vi "Controller Generate Filter Coefficients From Transfer Function.vi"(4 "Destination Folder":path, 5 "iwl coeff b":i16=2, 6 "Filter Name":string, 7 "iwl coeff a":i16=2, 8 "Generate FPGA Code?":bool, 9 "wl":i16=20, 10 "denominator":dbl[](array[numeric]), 11 "numerator":dbl[](array[numeric])) -> (1 "gain":dbl, 2 "coeff a":dbl[](array[numeric]), 3 "coeff b":dbl[](array[numeric]))   [LabVIEW 2011, in "Controller VIs.lvlib"]
uses:
  Controller VIs.lvlib
  <vilib>/addons/Digital Filter Design/_Objects.llb/DFD Output Iwl Obj.ctl
  <vilib>/addons/Digital Filter Design/_Objects.llb/DFD Quantization Settings.ctl
  <vilib>/addons/Digital Filter Design/_Objects.llb/DFD Quantization Sources.ctl
  <vilib>/addons/Digital Filter Design/_Objects.llb/DFD Phase Setting.ctl
  <vilib>/addons/Digital Filter Design/_Objects.llb/DFD Coef Norm Type.ctl
  <vilib>/addons/Digital Filter Design/FXPModel.llb/DFD FXP Quantize Coef (Advanced).vi
  <vilib>/addons/Digital Filter Design/NI_DigFilterLicensed.lvlib
  <vilib>/addons/Digital Filter Design/CodeGen.llb/DFD FXP LabVIEW FPGA Code Generator.vi
panel:
  out "max gain error (dB)":dbl
  out "max phase error (deg)":dbl
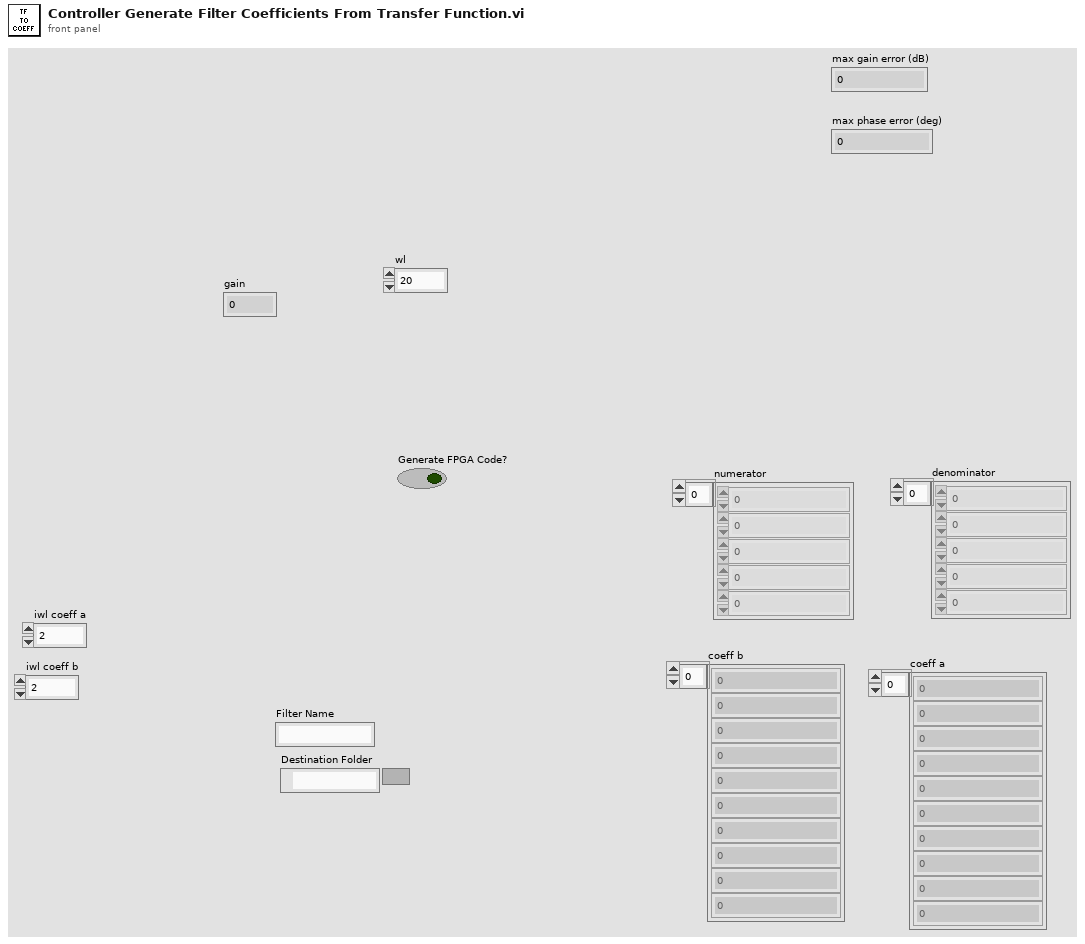
[diagram p1: front panel]
types:
  T1 = typedef "NI_DigFilterLicensed.lvlib/DFD Coef Norm Type.ctl" = enum16{"No Norm", "Time Domain 1-Norm", "Time Domain 2-Norm", "Time Domain Inf-Norm"}
  T2 = typedef "NI_DigFilterLicensed.lvlib/DFD Phase Setting.ctl" = cluster{"unwrap? (F)":bool, "degree? (F)":bool}
  T3 = typedef "NI_DigFilterLicensed.lvlib/DFD Quantization Settings.ctl" = cluster{"source":T4, "wl":i16, "iwl":i16, "overflow mode":enum16{"Saturation", "Wrap"}, "rounding mode":enum16{"Nearest", "Truncation"}, "signed?":bool}
  T4 = typedef "NI_DigFilterLicensed.lvlib/DFD Quantization Sources.ctl" = u16
  T5 = typedef "NI_DigFilterLicensed.lvlib/DFD Output Iwl Obj.ctl" = cluster{"output option":enum16{"Auto", "Same As Input", "User Defined"}, "integer word length":i16}
  T6 = typedef "NI_DigFilterLicensed.lvlib/DFD Filter Obj.ctl" = cluster{"mSRate_Fs":dbl, "mSRate_Version":string, "mSRate_Comments":string, "mSRate_OrgCoef":T7, "mSRate_CurCoef":T7, "mSRate_Quantized?":bool, "mSRate_QCoef":T7, "mSRate_QSettings":T9[], "mSRate_Order":i32, "mSRate_Scaling":cluster{"mSRate_ScaleByPowerOf2?":bool, "mSRate_ScaleType":T1}}
  T7 = typedef "NI_DigFilterLicensed.lvlib/DFD Filter Coef.ctl" = cluster{"type":T8, "gain":dbl, "coef a (k)":dbl[], "coef b (v)":dbl[]}
  T8 = typedef "NI_DigFilterLicensed.lvlib/DFD Filter Structure Type Selector.ctl" = enum16{"Undefined", "FIR Direct Form", "FIR Direct Form Transposed", "FIR Symmetric", "FIR Antisymmetric", "IIR Direct Form I", "IIR Direct Form I Transposed", "IIR Direct Form II", "IIR Direct Form II Transposed", "IIR Cascaded Second Order Sections Form I", "IIR Cascaded Second Order Sections Form I Transposed", "IIR Cascaded Second Order Sections Form II", "IIR Cascaded Second Order Sections Form II Transposed", "Lattice Allpass (basic sections)", "Lattice Allpass (one multiplier sections)", "Lattice Allpass (normalized sections)", "Lattice AR (basic sections)", "Lattice AR (one multiplier sections)", "Lattice AR (normalized sections)", "Lattice MA (minimum phase)", "Lattice MA (maximum phase)", "Lattice ARMA (basic sections)", "Lattice ARMA (one multiplier sections)", "Lattice ARMA (normalized sections)"}
  T9 = typedef "NI_DigFilterLicensed.lvlib/dfd_Internal Quantization Settings.ctl" = cluster{"source":T10, "wl":i16, "iwl":i16, "overflow mode":enum16{"Saturation", "Wrap"}, "rounding mode":enum16{"Nearest", "Truncation"}, "signed?":bool}
  T10 = typedef "NI_DigFilterLicensed.lvlib/dfd_Internal Quantization Srcs.ctl" = u16
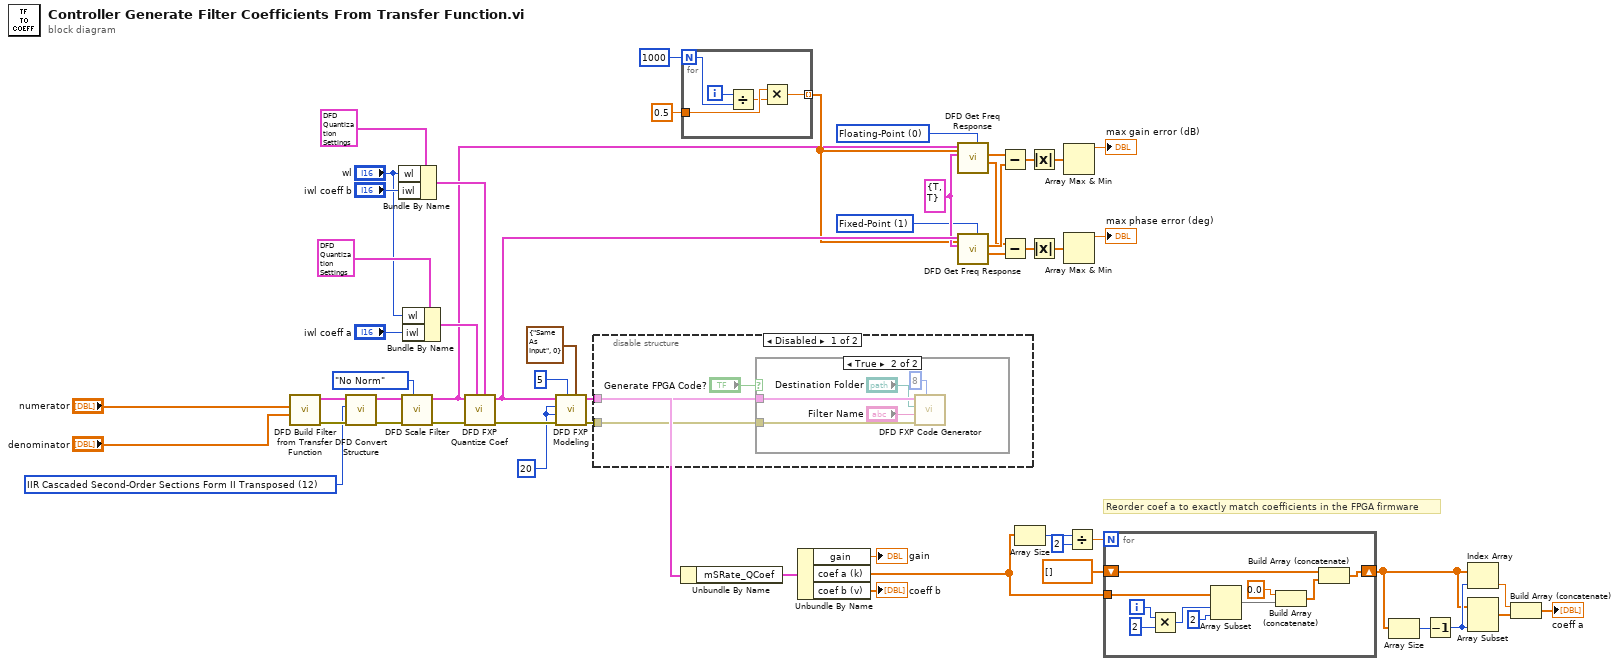
[diagram p0: block diagram]
diagram:
  w32 = u16 0 items=["Floating-Point", "Fixed-Point"] ("output option")
  w40 = u16 1 items=["Floating-Point", "Fixed-Point"] ("output option")
  w41 = T2 {"unwrap? (F)"=TRUE, "degree? (F)"=TRUE} ("phase view")
  w45 = i16 20 ("input word length")
  w52 = u16 12 items=["FIR Direct Form"=1, "FIR Direct Form Transposed"=2, "FIR Symmetric"=3, "FIR Antisymmetric"=4, "IIR Direct Form I"=5, "IIR Direct Form I Transposed"=6, "IIR Direct Form II"=7, "IIR Direct Form II Transposed"=8, "IIR Cascaded Second-Order Sections Form I"=9, "IIR Cascaded Second-Order Sections Form I Transposed"=10, "IIR Cascaded Second-Order Sections Form II"=11, "IIR Cascaded Second-Order Sections Form II Transposed"=12, "Lattice Allpass (basic sections)"=13, "Lattice Allpass (one multiplier sections)"=14, "Lattice Allpass (normalized sections)"=15, "Lattice AR (basic sections)"=16, "Lattice AR (one multiplier sections)"=17, "Lattice AR (normalized sections)"=18, "Lattice MA (minimum phase)"=19, "Lattice MA (maximum phase)"=20, "Lattice ARMA (basic sections)"=21, "Lattice ARMA (one multiplier sections)"=22, "Lattice ARMA (normalized sections)"=23] ("target structure")
  # "Reorder coef a to exactly match coefficients in the FPGA firmware"
  n1 = call <vilib>:"DFD Build Filter from Transfer Function.vi"("denominator"="denominator", "numerator"="numerator") -> ("error out"=w53:errorcluster, "filter out"=w47:T6)  [unwired: 8 in]
  n2 = call <vilib>:"DFD Convert Structure.vi"("error in (no error)"=w53, "target structure"=w52, "filter in"=w47) -> ("error out"=w18:errorcluster, "filter out"=w19:T6)  [unwired: 7 in]
  n3 = Bundle By Name(cluster=T3 {"source"=7, "wl"=20, "iwl"=1, "overflow mode"=enum."Saturation", "rounding mode"=enum."Nearest", "signed?"=TRUE} ("coefficients b/v quantizer"), "wl"="wl", "iwl"="iwl coeff b") -> (w34:T3)
  n4 = call <vilib>:"DFD Scale Filter.vi"("scale type"=DFD_Coef_Norm_Type."No Norm", "error in (no error)"=w18, "filter in"=w19) -> ("error out"=w17:errorcluster, "filter out"=w16:T6)  [unwired: 7 in]
  n5 = Bundle By Name(cluster=T3 {"source"=0, "wl"=20, "iwl"=1, "overflow mode"=enum."Saturation", "rounding mode"=enum."Nearest", "signed?"=TRUE} ("coefficients a/k quantizer"), "wl"="wl", "iwl"="iwl coeff a") -> (w33:T3)
  n6 = call-poly <vilib>:"DFD FXP Quantize Coef.vi"("coefficients b/v quantizer"=w34, "coefficients a/k quantizer"=w33, "error in (no error)"=w17, "filter in"=w16) -> ("error out"=w51:errorcluster, "filter out"=w42:T6)  [unwired: 6 in]
  n7 = call <vilib>:"DFD FXP Modeling.vi"("output integer word length"=T5 {"output option"=enum."Same As Input", "integer word length"=0}, "input integer word length"=i16 5, "error in (no error)"=w51, "output word length"=w45, "input word length"=w45, "filter in"=w42) -> ("error out"=w54:errorcluster, "filter out"=w43:T6)  [unwired: 4 in]
  n8 = disable-structure shown="Disabled" {
    disable-tunnel: w54 -> [w57 _]
    disable-tunnel: w43 -> [w56 _]
    frame Disabled {
      n9 = case shown="True" "Generate FPGA Code?" {
        tunnel: w57 -> [_ w62]
        tunnel: w56 -> [_ w61]
        frame False {
        }
        frame True {
          n10 = call-poly <vilib>:"DFD FXP Code Generator.vi"("# channels"=8, "error in (no error)"=w62, "filter name"="Filter Name", "destination folder"="Destination Folder", "filter in"=w61) -> ()  [unwired: 2 in, 5 out]
        }
      }
    }
    frame Enabled {
    }
  }
  n11 = Unbundle By Name(w43) -> ("mSRate_QCoef"=w50:T7)
  n12 = for {
    N: 1000 -> [w66]
    tunnel: 0.5 -> [w65]
    tunnel: [w63] -> w27 mode=indexing
    i -> [w67]
    n13 = Divide(x=w67, y=w66) -> (x/y=w64:dbl)
    n14 = Multiply(x=w65, y=w64) -> (x*y=w63:dbl)
  }
  n15 = Unbundle By Name(w50) -> ("gain"=→"gain":dbl, "coef a (k)"=w11:dbl[], "coef b (v)"=→"coeff b":dbl[])
  n16 = call <vilib>:"DFD Get Freq Response.vi"("output option"=w32, "freq points [Hz]"=w27, "phase view"=w41, "filter in"=w16) -> ("phase"=w29:dbl[], "magnitude"=w31:dbl[])  [unwired: 4 in, 2 out]
  n17 = call <vilib>:"DFD Get Freq Response.vi"("output option"=w40, "freq points [Hz]"=w27, "phase view"=w41, "filter in"=w42) -> ("phase"=w28:dbl[], "magnitude"=w30:dbl[])  [unwired: 4 in, 2 out]
  n18 = Subtract(x=w31, y=w30) -> (x-y=w25:dbl[])
  n19 = Subtract(x=w29, y=w28) -> (x-y=w22:dbl[])
  n20 = Array Size(array=w11) -> (size(s)=w10:i32)
  n21 = Absolute Value(x=w25) -> (abs(x)=w24:dbl[])
  n22 = Absolute Value(x=w22) -> (abs(x)=w23:dbl[])
  n23 = Array Max & Min(array=w24) -> (max value=→"max gain error (dB)":dbl)  [unwired: 3 out]
  n24 = Array Max & Min(array=w23) -> (max value=→"max phase error (deg)":dbl)  [unwired: 3 out]
  n25 = Divide(x=w10, y=2) -> (x/y=w13:dbl)
  n26 = for {
    N: w13 -> [_]
    tunnel: w11 -> [w70]
    shift-right: [w68] -> w5
    shift-left: dbl[] [] ("coef a (k)") -> [w69]
    i -> [w77]
    n27 = Multiply(x=w77, y=2) -> (x*y=w75:i32)
    n28 = Array Subset(array=w70, index=w75, length=2) -> (w73:dbl[])
    n29 = Build Array (concatenate)(0.0 ("x/y"), w73) -> (w71:dbl[])
    n30 = Build Array (concatenate)(w69, w71) -> (w68:dbl[])
  }
  n31 = Array Size(array=w5) -> (size(s)=w4:i32)
  n32 = Decrement(x=w4) -> (x-1=w8:i32)
  n33 = Index Array(array=w5, index=w8) -> (element=w7:dbl)
  n34 = Array Subset(array=w5, length=w8) -> (w6:dbl[])  [unwired: 1 in]
  n35 = Build Array (concatenate)(w7, w6) -> (→"coeff a":dbl[])
